vi "CRYDB Insert Into UnitTable.vi"(0 "connection reference":T2, 1 "Unit_Abbreviation":string, 2 "Unit Name":string, 3 "error in":errorcluster) -> (7 "connection reference out":T2, 8 "Unit ID":i32, 10 "error out":errorcluster)   [LabVIEW 2013]
uses:
  <vilib>/addons/database/Connection.llb/Conn ObjectReference.ctl
  <vilib>/addons/database/Auxilliary.llb/DB Tools Column Info.ctl
  <vilib>/addons/database/Auxilliary.llb/DB Tools DataTypes.ctl
  <vilib>/addons/database/Connection.llb/Conn Execute.vi
  <vilib>/addons/database/Recordset.llb/Rec Fetch Recordset Data (R).vi
  <vilib>/addons/database/Recordset.llb/Rec Destroy - Connection.vi
  <vilib>/addons/database/_DB Variant To Data/Database Variant To Data.xnode
  <vilib>/addons/database/NI_Database_API.lvlib
panel:
  in  "Table":T1
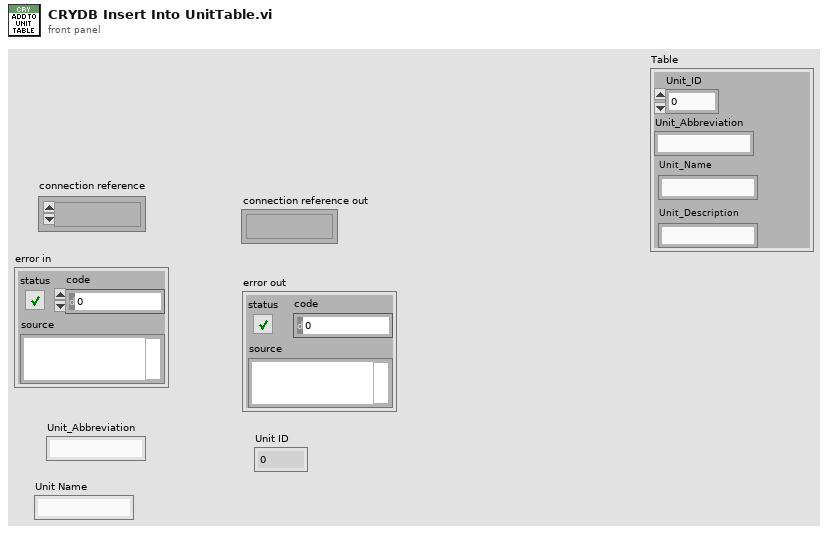
[diagram p1: front panel]
types:
  T1 = cluster{"Unit_ID":u32, "Unit_Abbreviation":string, "Unit_Name":string, "Unit_Description":string}
  T2 = typedef "NI_Database_API.lvlib/Conn ObjectReference.ctl" = refnum<k1>
  T3 = typedef "NI_Database_API.lvlib/DB Tools Column Info.ctl" = cluster{"column name":string, "data type":T4, "size":i32, "allow null?":bool}
  T4 = typedef "NI_Database_API.lvlib/DB Tools DataTypes.ctl" = enum16{"String", "Long (I32)", "Single (SGL)", "Double (DBL)", "Date/Time", "Binary"}
  T5 = typedef "NI_Database_API.lvlib/Rec ObjectReference.ctl" = refnum<k1>
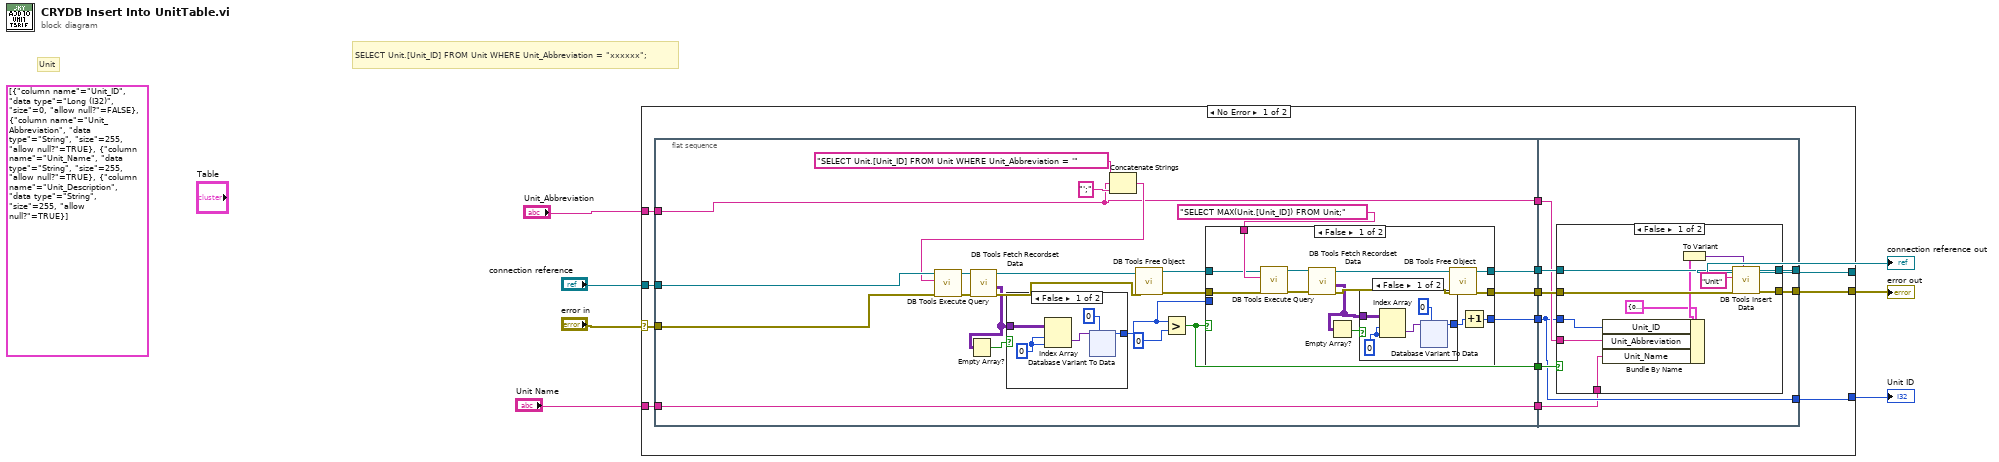
[diagram p0: block diagram]
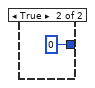
[diagram p2: hidden frame]
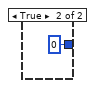
[diagram p3: hidden frame]
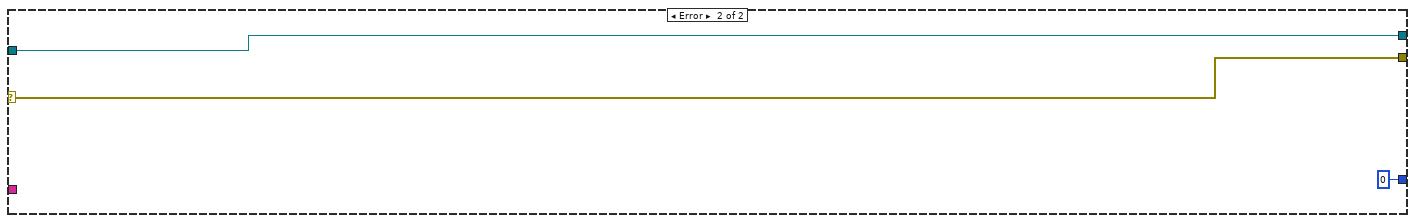
[diagram p6: hidden frame]
diagram:
  (unwired) T3[] [{"column name"="Unit_ID", "data type"=enum."Long (I32)", "size"=0, "allow null?"=FALSE}, {"column name"="Unit_Abbreviation", "data type"=enum."String", "size"=255, "allow null?"=TRUE}, {"column name"="Unit_Name", "data type"=enum."String", "size"=255, "allow null?"=TRUE}, {"column name"="Unit_Description", "data type"=enum."String", "size"=255, "allow null?"=TRUE}] ("column information")
  # "Unit"
  # "SELECT Unit.[Unit_ID] FROM Unit WHERE Unit_Abbreviation = \"xxxxxx\";"
  n1 = case shown="No Error" "error in" {
    selector: "error in" -> [w18 w157]
    tunnel: "connection reference" -> [w20 w158]
    tunnel: [w16 w158] -> w4
    tunnel: [w15 w157] -> w5
    tunnel: [w11 0 ("data")] -> w3
    tunnel: "Unit_Abbreviation" -> [w10 _]
    tunnel: "Unit Name" -> [w9 _]
    frame No Error {
      n2 = flat-sequence {
        tunnel: w20 -> [w42]
        tunnel: [w29] -> w19
        tunnel: w18 -> [w38]
        tunnel: [w28] -> w17
        tunnel: [w27] -> w14
        tunnel: [w26] -> w13
        tunnel: [w25] -> w12
        tunnel: w10 -> [w25]
        tunnel: w9 -> [w24]
        tunnel: [w24] -> w8
        tunnel: w19 -> [w142]
        tunnel: w17 -> [w141]
        tunnel: [w140] -> w16
        tunnel: [w139] -> w15
        tunnel: w14 -> [w138]
        tunnel: w13 -> [w136]
        tunnel: w12 -> [w137]
        tunnel: [w136] -> w11
        tunnel: w8 -> [w135]
        frame #0 {
          n3 = Concatenate Strings("SELECT Unit.[Unit_ID] FROM Unit WHERE Unit_Abbreviation = '" ("SQL query"), w25, "';" ("string")) -> (w33:string)
          n4 = call-poly <vilib>:"DB Tools Execute Query.vi"("error in (no error)"=w38, "SQL query"=w33, "connection reference"=w42) -> ("error out"=w37:errorcluster, "recordset reference"=w41:T5)  [unwired: 5 in]
          n5 = call-poly <vilib>:"DB Tools Fetch Recordset Data.vi"("error in (no error)"=w37, "recordset reference"=w41) -> ("error out"=w36:errorcluster, "recordset data"=w21:variant[][], "recordset reference out"=w40:T5)  [unwired: 3 in]
          n6 = Empty Array?(array=w21) -> (empty?=w23:bool)
          n7 = case shown="False" w23 {
            tunnel: w21 -> [w47 _]
            tunnel: [w44 0 ("data")] -> w22
            frame False {
              w46 = 0 ("disabled index (col)")
              n8 = Index Array(array=w47, index (row)=w46, index (col)=w46) -> (element=w43:variant)
              n9 = xnode "Database Variant To Data"("database variant"=w43, "type"=0) -> ("data"=w44:i32)  [unwired: 1 in, 1 out]
            }
            frame True {
            }
          }
          n10 = call-poly <vilib>:"DB Tools Free Object.vi"("error in (no error)"=w36, "recordset reference"=w40) -> ("error out"=w31:errorcluster, "connection reference"=w32:T2)  [unwired: 8 in]
          n11 = Greater?(x=w22, y=0) -> (0:w27:bool)
          n12 = case shown="False" w27 {
            tunnel: w22 -> [_ w134]
            tunnel: w32 -> [w92 w133]
            tunnel: w31 -> [w91 w132]
            tunnel: "SELECT MAX(Unit.[Unit_ID]) FROM Unit;" ("SQL query") -> [w93 _]
            tunnel: [w88 w134] -> w26
            tunnel: [w85 w133] -> w29
            tunnel: [w84 w132] -> w28
            frame False {
              n13 = call-poly <vilib>:"DB Tools Execute Query.vi"("error in (no error)"=w91, "SQL query"=w93, "connection reference"=w92) -> ("error out"=w89:errorcluster, "recordset reference"=w90:T5)  [unwired: 5 in]
              n14 = call-poly <vilib>:"DB Tools Fetch Recordset Data.vi"("error in (no error)"=w89, "recordset reference"=w90) -> ("error out"=w86:errorcluster, "recordset data"=w81:variant[][], "recordset reference out"=w87:T5)  [unwired: 3 in]
              n15 = Empty Array?(array=w81) -> (empty?=w83:bool)
              n16 = case shown="False" w83 {
                tunnel: w81 -> [w98 _]
                tunnel: [w95 0 ("data")] -> w82
                frame False {
                  w97 = 0 ("disabled index (col)")
                  n17 = Index Array(array=w98, index (row)=w97, index (col)=w97) -> (element=w94:variant)
                  n18 = xnode "Database Variant To Data"("database variant"=w94, "type"=0) -> ("data"=w95:i32)  [unwired: 1 in, 1 out]
                }
                frame True {
                }
              }
              n19 = call-poly <vilib>:"DB Tools Free Object.vi"("error in (no error)"=w86, "recordset reference"=w87) -> ("error out"=w84:errorcluster, "connection reference"=w85:T2)  [unwired: 8 in]
              n20 = Increment(x=w82) -> (x+1=w88:i32)
            }
            frame True {
            }
          }
        }
        frame #1 {
          n21 = case shown="False" w138 {
            tunnel: w142 -> [w153 w155]
            tunnel: w141 -> [w151 w154]
            tunnel: [w149 w155] -> w140
            tunnel: [w148 w154] -> w139
            tunnel: w136 -> [w147 _]
            tunnel: w137 -> [w146 _]
            tunnel: w135 -> [w143 _]
            frame False {
              n22 = Bundle By Name(cluster=T1 {"Unit_ID"=0, "Unit_Abbreviation"="", "Unit_Name"="", "Unit_Description"=""} ("Table"), "Unit_ID"=w147, "Unit_Abbreviation"=w146, "Unit_Name"=w143) -> (w145:T1)
              n23 = To Variant(anything=w145) -> (Variant=w150:variant)
              n24 = call <vilib>:"DB Tools Insert Data.vi"("data"=w150, "error in (no error)"=w151, "table"="Unit", "connection reference"=w153) -> ("error out"=w148:errorcluster, "connection reference out"=w149:T2)  [unwired: 6 in]
            }
            frame True {
            }
          }
        }
      }
    }
    frame Error {
    }
  }
  "connection reference out" <- w4
  "error out" <- w5
  "Unit ID" <- w3
